vi "Oscillate.vi"(10 "Target In Sight?":bool, 11 "Effort":dbl=0.25 format="%#_13g") -> ()   [LabVIEW 2016]
uses:
  Systems/Global 1.vi
panel:
  in  "ampliture":i32=2000
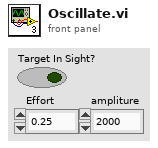
[diagram p1: front panel]
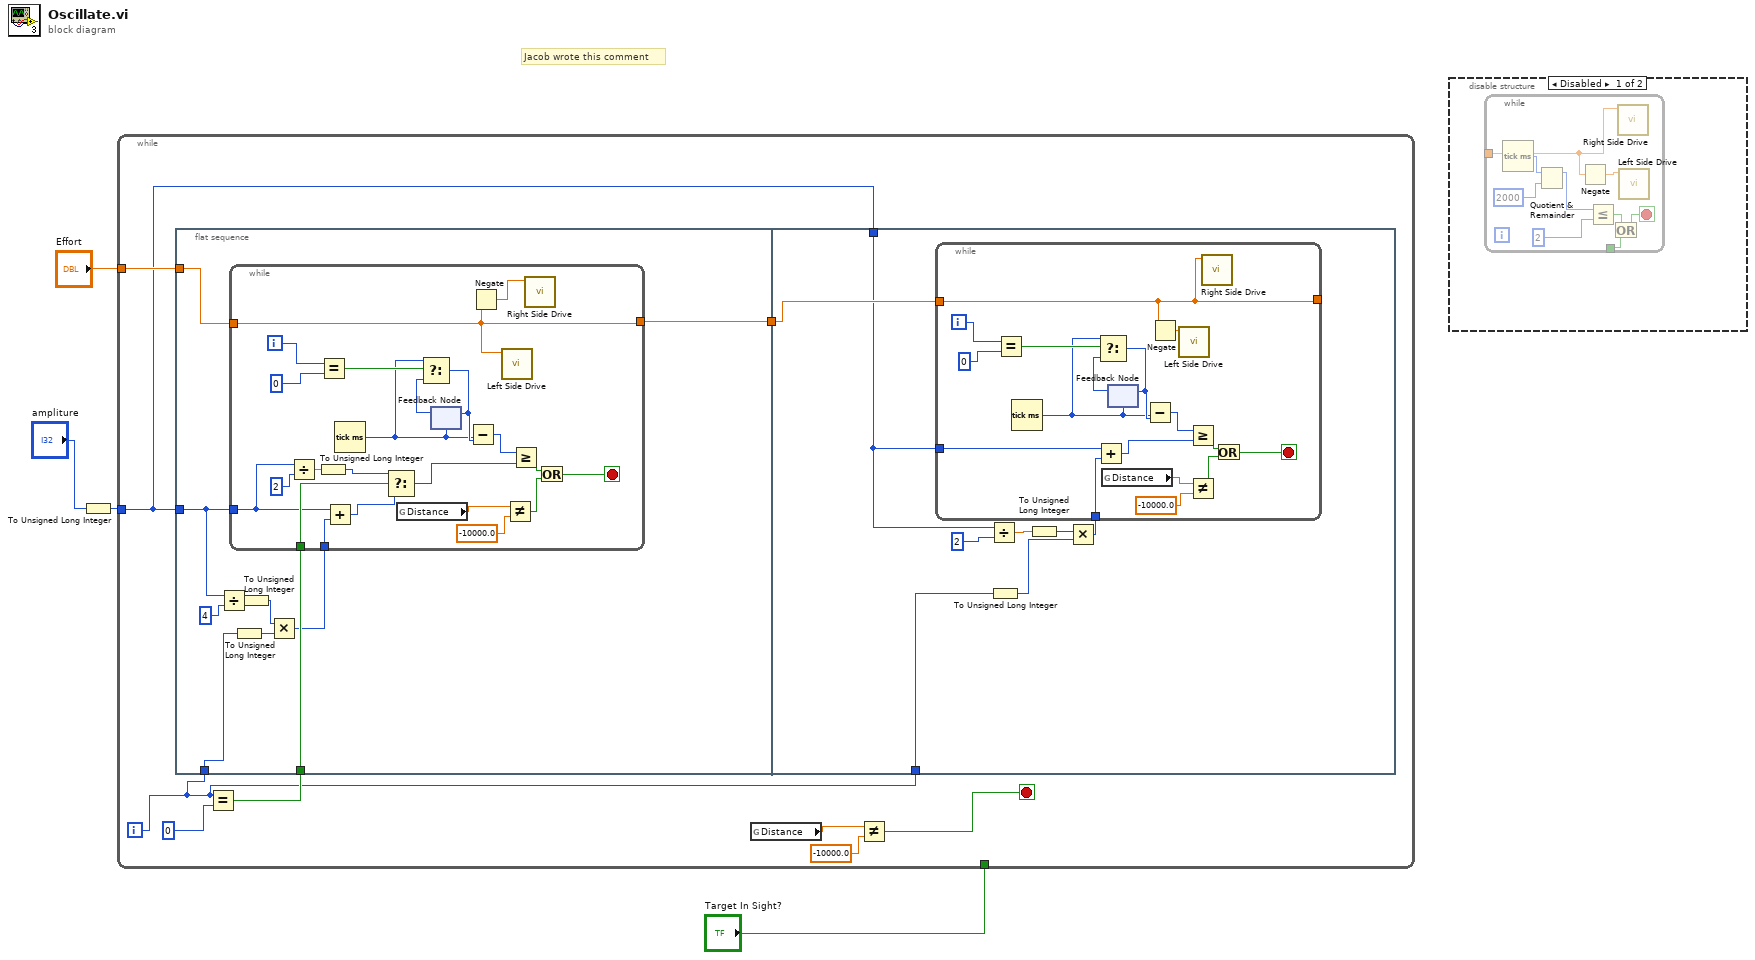
[diagram p0: block diagram]
diagram:
  # "Jacob wrote this comment"
  n1 = To Unsigned Long Integer(number="ampliture") -> (unsigned 32bit integer=w1:u32)
  n2 = while {
    tunnel: "Target In Sight?" -> [_]
    tunnel: "Effort" -> [w13]
    tunnel: w1 -> [w8]
    i -> [w9]
    stop <- w5 stop-if-true
    n3 = flat-sequence {
      tunnel: w13 -> [w23]
      tunnel: [w22] -> w12
      tunnel: w10 -> [w21]
      tunnel: w9 -> [w19]
      tunnel: w8 -> [w17]
      tunnel: w12 -> [w53]
      tunnel: w9 -> [w50]
      tunnel: w8 -> [w46]
      frame #0 {
        n4 = Divide(x=w17, y=u32 4 ("milliseconds to wait")) -> (x/y=w16:dbl)
        n5 = To Unsigned Long Integer(number=w19) -> (unsigned 32bit integer=w18:u32)
        n6 = To Unsigned Long Integer(number=w16) -> (unsigned 32bit integer=w14:u32)
        n7 = Multiply(x=w14, y=w18) -> (x*y=w20:u32)
        n8 = while {
          tunnel: w23 -> [w44]
          tunnel: [w44] -> w22
          tunnel: w21 -> [w33]
          tunnel: w20 -> [w31]
          tunnel: w17 -> [w29]
          i -> [w39]
          stop <- w45 stop-if-true
          n9 = Divide(x=w29, y=u32 2 ("milliseconds to wait")) -> (x/y=w30:dbl)
          n10 = To Unsigned Long Integer(number=w30) -> (unsigned 32bit integer=w27:u32)
          n11 = Equal?(x=w39, y=0) -> (x = y?=w37:bool)
          n12 = Add(x=w29, y=w31) -> (x+y=w32:u32)
          n13 = Tick Count (ms)() -> (millisecond timer value=w35:u32)
          n14 = Select(t=w27, s=w33, f=w32) -> (s? t:f=w34:u32)
          n15 = global read "Global 1.vi" "Distance"() -> (w26:dbl)
          n16 = feedback #1(w35) -> (w36:u32)
          n17 = Select(t=w35, s=w37, f=w36) -> (s? t:f=w40:u32)
          n18 = feedback-in #1(w40) -> ()
          n19 = Subtract(x=w35, y=w40) -> (x-y=w42:u32)
          n20 = Negate(x=w44) -> (-x=w43:dbl)
          n21 = call "Left Side Drive.vi"("Effort"=w44) -> ()  [unwired: 11 in]
          n22 = Not Equal?(x=w26, y=-10000.0) -> (x != y?=w24:bool)
          n23 = Greater Or Equal?(x=w42, y=w34) -> (x >= y?=w41:bool)
          n24 = call "Right Side Drive.vi"("Effort"=w43) -> ()  [unwired: 11 in]
          n25 = Or(x=w41, y=w24) -> (x .or. y?=w45:bool)
        }
      }
      frame #1 {
        n26 = Divide(x=w46, y=u32 2 ("milliseconds to wait")) -> (x/y=w48:dbl)
        n27 = To Unsigned Long Integer(number=w50) -> (unsigned 32bit integer=w52:u32)
        n28 = To Unsigned Long Integer(number=w48) -> (unsigned 32bit integer=w47:u32)
        n29 = Multiply(x=w47, y=w52) -> (x*y=w51:u32)
        n30 = while {
          tunnel: w53 -> [w61]
          tunnel: [w61] -> _
          tunnel: w51 -> [w59]
          tunnel: w46 -> [w57]
          i -> [w66]
          stop <- w70 stop-if-true
          n31 = Equal?(x=w66, y=0) -> (x = y?=w64:bool)
          n32 = Tick Count (ms)() -> (millisecond timer value=w62:u32)
          n33 = Add(x=w57, y=w59) -> (x+y=w58:u32)
          n34 = global read "Global 1.vi" "Distance"() -> (w55:dbl)
          n35 = feedback #2(w62) -> (w63:u32)
          n36 = Select(t=w62, s=w64, f=w63) -> (s? t:f=w67:u32)
          n37 = feedback-in #2(w67) -> ()
          n38 = Subtract(x=w62, y=w67) -> (x-y=w69:u32)
          n39 = Negate(x=w61) -> (-x=w60:dbl)
          n40 = call "Left Side Drive.vi"("Effort"=w60) -> ()  [unwired: 11 in]
          n41 = Greater Or Equal?(x=w69, y=w58) -> (x >= y?=w68:bool)
          n42 = Not Equal?(x=w55, y=-10000.0) -> (x != y?=w54:bool)
          n43 = call "Right Side Drive.vi"("Effort"=w61) -> ()  [unwired: 11 in]
          n44 = Or(x=w68, y=w54) -> (x .or. y?=w70:bool)
        }
      }
    }
    n45 = Equal?(x=w9, y=0) -> (x = y?=w10:bool)
    n46 = global read "Global 1.vi" "Distance"() -> (w7:dbl)
    n47 = Not Equal?(x=w7, y=-10000.0) -> (x != y?=w5:bool)
  }
  n48 = disable-structure shown="Disabled" {
    frame Disabled {
      n49 = while {
        tunnel: _ -> [w78]
        tunnel: _ -> [w71]
        stop <- w72 stop-if-true
        n50 = Tick Count (ms)() -> (millisecond timer value=w75:u32)
        n51 = Quotient & Remainder(x=w75, y=u32 2000 ("milliseconds to wait")) -> (x-y*floor(x/y)=w74:u32)  [unwired: 1 out]
        n52 = Negate(x=w78) -> (-x=w79:dbl)
        n53 = Less Or Equal?(x=w74, y=u32 2 ("milliseconds to wait")) -> (x <= y?=w73:bool)
        n54 = Or(x=w73, y=w71) -> (x .or. y?=w72:bool)
        n55 = call "Right Side Drive.vi"("Effort"=w78) -> ()  [unwired: 11 in]
        n56 = call "Left Side Drive.vi"("Effort"=w79) -> ()  [unwired: 11 in]
      }
    }
    frame Enabled {
    }
  }
